vi "Write Setting_ver2.vi"(0 "configuration file path":path, 1 "output cluster":T1, 3 "error in (no error)":errorcluster) -> (7 "file path":path, 10 "error out":errorcluster)   [LabVIEW 2023]
uses:
  <vilib>/Utility/config.llb/Write Key (I32).vi
  <vilib>/Utility/config.llb/Write Key (Double).vi
  <vilib>/Utility/config.llb/Write Key (Path).vi
  <vilib>/Utility/config.llb/Write Key (String).vi
  <vilib>/Utility/config.llb/Write Key (U32).vi
  <vilib>/Utility/config.llb/NI_LVConfig.lvlib
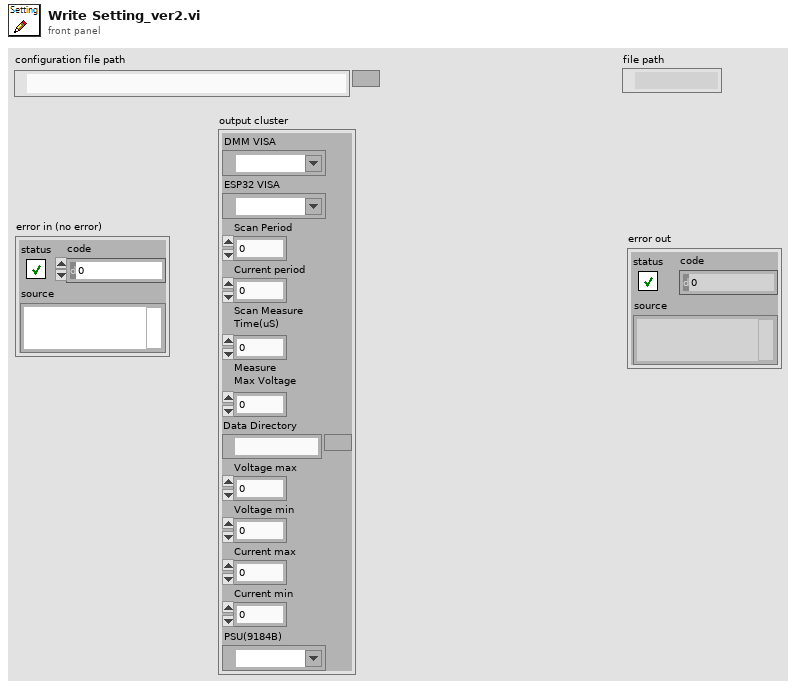
[diagram p1: front panel]
types:
  T1 = cluster{"DMM VISA":refnum<visa-resource-name>, "ESP32 VISA":refnum<visa-resource-name>, "Scan Period":u32, "Current period":u32, "Scan Measure\nTime(uS)":i32, "Measure\nMax Voltage":dbl, "Data Directory":path, "Voltage max":dbl, "Voltage min":dbl, "Current max":dbl, "Current min":dbl, "PSU(9184B)":refnum<visa-resource-name>}
  T2 = typedef "NI_LVConfig.lvlib/Config Data RefNum.ctl" = refnum<k1>
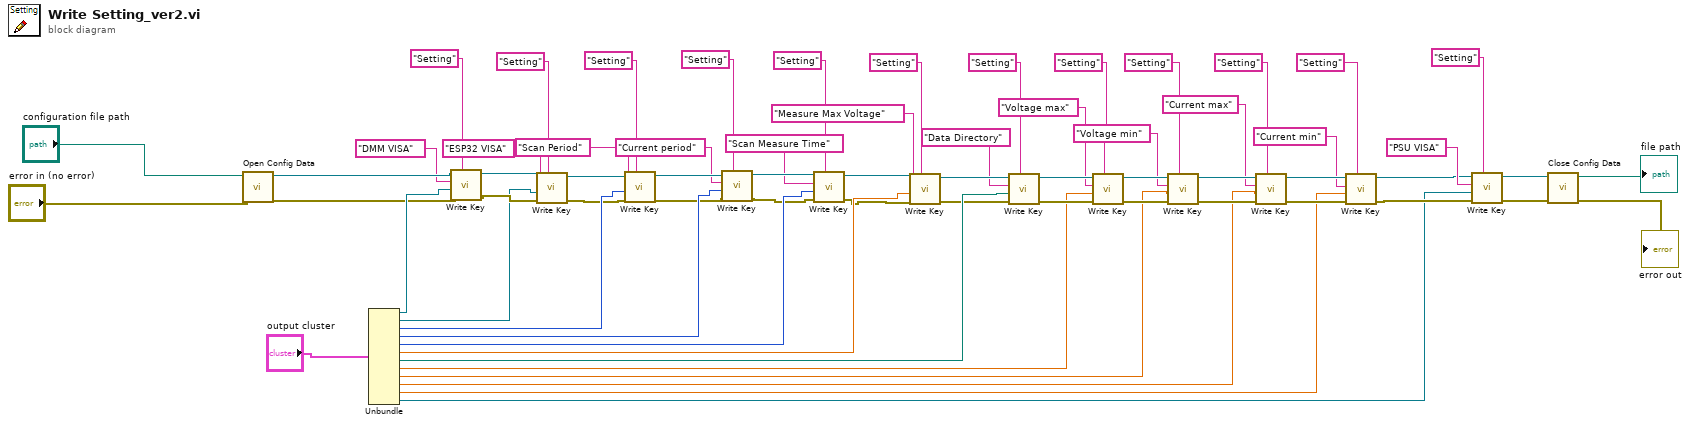
[diagram p0: block diagram]
diagram:
  n1 = call <vilib>:"Open Config Data.vi"("error in (no error)"="error in (no error)", "configuration file path"="configuration file path") -> ("error out"=w49:errorcluster, "refnum"=w50:T2)  [unwired: 7 in, 1 out]
  n2 = Unbundle("output cluster") -> ("DMM VISA"=w62:refnum<visa-resource-name>, "ESP32 VISA"=w35:refnum<visa-resource-name>, "Scan Period"=w56:u32, "Current period"=w55:u32, "Scan Measure\nTime(uS)"=w54:i32, "Measure\nMax Voltage"=w53:dbl, "Data Directory"=w51:path, "Voltage max"=w15:dbl, "Voltage min"=w14:dbl, "Current max"=w13:dbl, "Current min"=w12:dbl, "PSU(9184B)"=w1:refnum<visa-resource-name>)
  n3 = call-poly <vilib>:"Write Key.vi"("section"="Setting", "error in (no error)"=w49, "value"=w62, "key"="DMM VISA", "refnum"=w50) -> ("error out"=w37:errorcluster, "refnum out"=w48:T2)  [unwired: 4 in, 1 out]
  n4 = call-poly <vilib>:"Write Key.vi"("section"="Setting", "error in (no error)"=w37, "value"=w35, "key"="ESP32 VISA", "refnum"=w48) -> ("error out"=w46:errorcluster, "refnum out"=w47:T2)  [unwired: 4 in, 1 out]
  n5 = call-poly <vilib>:"Write Key.vi"("section"="Setting", "error in (no error)"=w46, "value"=w56, "key"="Scan Period", "refnum"=w47) -> ("error out"=w44:errorcluster, "refnum out"=w45:T2)  [unwired: 4 in, 1 out]
  n6 = call-poly <vilib>:"Write Key.vi"("section"="Setting", "error in (no error)"=w44, "value"=w55, "key"="Current period", "refnum"=w45) -> ("error out"=w42:errorcluster, "refnum out"=w43:T2)  [unwired: 4 in, 1 out]
  n7 = call-poly <vilib>:"Write Key.vi"("section"="Setting", "error in (no error)"=w42, "value"=w54, "key"="Scan Measure Time", "refnum"=w43) -> ("error out"=w40:errorcluster, "refnum out"=w41:T2)  [unwired: 4 in, 1 out]
  n8 = call-poly <vilib>:"Write Key.vi"("section"="Setting", "error in (no error)"=w40, "value"=w53, "key"="Measure Max Voltage", "refnum"=w41) -> ("error out"=w38:errorcluster, "refnum out"=w39:T2)  [unwired: 4 in, 1 out]
  n9 = call-poly <vilib>:"Write Key.vi"("section"="Setting", "error in (no error)"=w38, "value"=w51, "key"="Data Directory", "refnum"=w39) -> ("error out"=w28:errorcluster, "refnum out"=w21:T2)  [unwired: 4 in, 1 out]
  n10 = call-poly <vilib>:"Write Key.vi"("section"="Setting", "error in (no error)"=w28, "value"=w15, "key"="Voltage max", "refnum"=w21) -> ("error out"=w26:errorcluster, "refnum out"=w27:T2)  [unwired: 4 in, 1 out]
  n11 = call-poly <vilib>:"Write Key.vi"("section"="Setting", "error in (no error)"=w26, "value"=w14, "key"="Voltage min", "refnum"=w27) -> ("error out"=w24:errorcluster, "refnum out"=w25:T2)  [unwired: 4 in, 1 out]
  n12 = call-poly <vilib>:"Write Key.vi"("section"="Setting", "error in (no error)"=w24, "value"=w13, "key"="Current max", "refnum"=w25) -> ("error out"=w22:errorcluster, "refnum out"=w23:T2)  [unwired: 4 in, 1 out]
  n13 = call-poly <vilib>:"Write Key.vi"("section"="Setting", "error in (no error)"=w22, "value"=w12, "key"="Current min", "refnum"=w23) -> ("error out"=w4:errorcluster, "refnum out"=w5:T2)  [unwired: 4 in, 1 out]
  n14 = call-poly <vilib>:"Write Key.vi"("section"="Setting", "error in (no error)"=w4, "value"=w1, "key"="PSU VISA", "refnum"=w5) -> ("error out"=w2:errorcluster, "refnum out"=w3:T2)  [unwired: 4 in, 1 out]
  n15 = call <vilib>:"Close Config Data.vi"("error in (no error)"=w2, "refnum"=w3) -> ("error out"=→"error out":errorcluster, "file path"=→"file path":path)  [unwired: 8 in]
